vi "Prepare_outputfiles.vi"(8 "error in":errorcluster, 10 "Dynamic data in":T1, 11 "Input parameters 2":T2={"Measurement type"=enum."Debug", "Sensor type"=enum."HPK_8in_256", "Identifier"="test.txt", "Open after execution?"=FALSE, "Plot after execution?"=FALSE, "Display channel"=0, "Voltage Delay (s)"=0.5, "Switch Delay (s)"=0.01, "VISA resource name source"="", "VISA resource name DMM"="", "VISA resource name LCR"="", "Compliance  Level (uA)"=10.0, "Voltage Limit (V)"=1000.0, "Data storage location"="", "Scan voltages"="", "Use source as DMM?"=FALSE, "LCR signal frequenzy (Hz)"=10.0, "DMM device"=enum."Keithley2001", "Sampling number"=1, "Use env. sensors on"=enum."Sensirion sht1x/7x", "Switchboard Handle"=0, "Use Switchboard"=FALSE, "LCR signal voltage (V)"=10000.0, "Repeat"=1, "Test Run Limit (nA)"=10.0, "Scan voltages IV"="", "Scan voltages CV"="", "Hex pad numbers?"=FALSE, "Set measurement type"=enum."Debug", "Custom pad scan"="", "IV voltage Delay (s)"=0.5, "CV voltage Delay (s)"=0.5} {"CV voltage Delay (s)" format="%#_13g"; "IV voltage Delay (s)" format="%#_13g"; "Voltage Limit (V)" format="%#_13g"; "Voltage Delay (s)" format="%#_13g"; "Switch Delay (s)" format="%#_13g"}) -> (0 "error out":errorcluster, 2 "Dynamic data out":T1, 3 "Input parameters":T2={"Measurement type"=enum."Debug", "Sensor type"=enum."HPK_8in_256", "Identifier"="test.txt", "Open after execution?"=FALSE, "Plot after execution?"=FALSE, "Display channel"=0, "Voltage Delay (s)"=0.5, "Switch Delay (s)"=0.01, "VISA resource name source"="", "VISA resource name DMM"="", "VISA resource name LCR"="", "Compliance  Level (uA)"=10.0, "Voltage Limit (V)"=1000.0, "Data storage location"="", "Scan voltages"="", "Use source as DMM?"=FALSE, "LCR signal frequenzy (Hz)"=10.0, "DMM device"=enum."Keithley2001", "Sampling number"=1, "Use env. sensors on"=enum."Sensirion sht1x/7x", "Switchboard Handle"=0, "Use Switchboard"=FALSE, "LCR signal voltage (V)"=10000.0, "Repeat"=1, "Test Run Limit (nA)"=10.0, "Scan voltages IV"="", "Scan voltages CV"="", "Hex pad numbers?"=FALSE, "Set measurement type"=enum."Debug", "Custom pad scan"="", "IV voltage Delay (s)"=0.5, "CV voltage Delay (s)"=0.5} {"CV voltage Delay (s)" format="%#_13g"; "IV voltage Delay (s)" format="%#_13g"; "Voltage Limit (V)" format="%#_13g"; "Voltage Delay (s)" format="%#_13g"; "Switch Delay (s)" format="%#_13g"})   [LabVIEW 2016]
uses:
  Input_parameters.ctl
  Dynamic_data.ctl
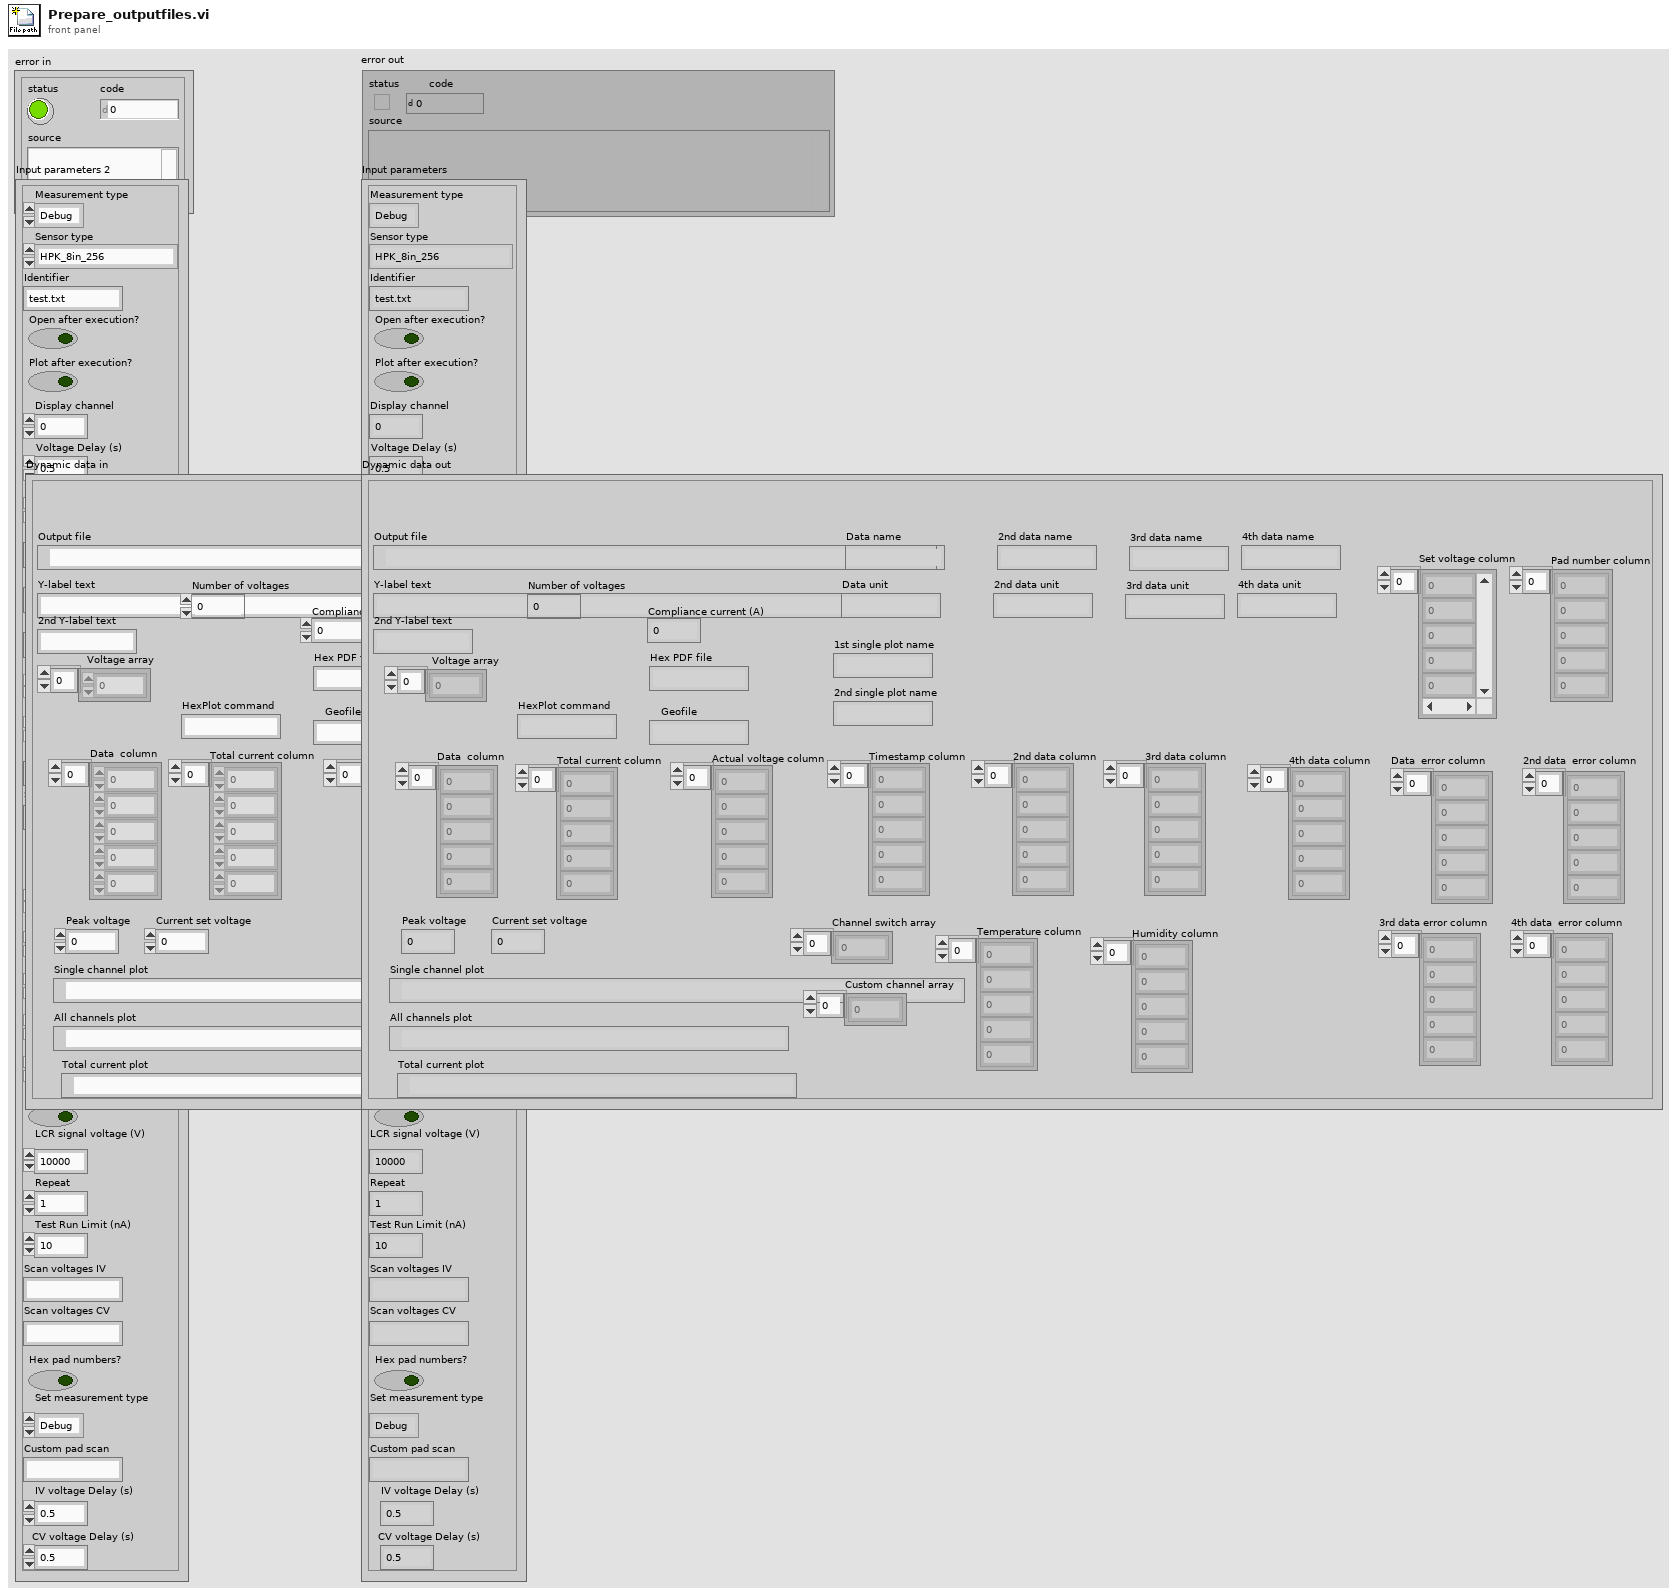
[diagram p1: front panel]
types:
  T1 = typedef "Dynamic_data.ctl" = cluster{"Output file":path, "Y-label text":string, "Current set voltage":dbl, "Set voltage column":dbl[], "Pad number column":dbl[], "Data  column":dbl[], "Number of voltages":i32, "Compliance current (A)":dbl, "Geofile":string, "Peak voltage":dbl, "Hex PDF file":string, "Voltage array":dbl[], "Total current column":dbl[], "Timestamp column":dbl[], "Data name":string, "Data unit":string, "2nd data column":dbl[], "2nd data name":string, "2nd data unit":string, "3rd data column":dbl[], "4th data column":dbl[], "3rd data name":string, "3rd data unit":string, "4th data name":string, "4th data unit":string, "Actual voltage column":dbl[], "2nd Y-label text":string, "Single channel plot":path, "Temperature column":dbl[], "Humidity column":dbl[], "Channel switch array":i32[], "1st single plot name":string, "2nd single plot name":string, "All channels plot":path, "HexPlot command":string, "Custom channel array":i32[], "Data  error column":dbl[], "2nd data  error column":dbl[], "3rd data error column":dbl[], "4th data  error column":dbl[], "Total current plot":path}
  T2 = typedef "Input_parameters.ctl" = cluster{"Measurement type":enum16{"IV", "CV", "Debug", "Test"}, "Sensor type":enum16{"HPK_6in_135", "HPK_8in_256", "INF_8in_256", "Diode", "HPK_6in_256", "Test capacitances", "Full matrix"}, "Identifier":string, "Open after execution?":bool, "Plot after execution?":bool, "Display channel":i32, "Voltage Delay (s)":dbl, "Switch Delay (s)":dbl, "VISA resource name source":refnum<visa-resource-name>, "VISA resource name DMM":refnum<visa-resource-name>, "VISA resource name LCR":refnum<visa-resource-name>, "Compliance  Level (uA)":dbl, "Voltage Limit (V)":dbl, "Data storage location":string, "Scan voltages":string, "Use source as DMM?":bool, "LCR signal frequenzy (Hz)":dbl, "DMM device":enum16{"Keithley2001", "Keithley2450", "Keithley2410", "Keithley6487"}, "Sampling number":i32, "Use env. sensors on":enum16{"Sensirion sht1x/7x", "Switch Matrix", "Probecard"}, "Switchboard Handle":u32, "Use Switchboard":bool, "LCR signal voltage (V)":dbl, "Repeat":i32, "Test Run Limit (nA)":dbl, "Scan voltages IV":string, "Scan voltages CV":string, "Hex pad numbers?":bool, "Set measurement type":enum16{"IV", "CV", "Debug", "Test", "IV+CV"}, "Custom pad scan":string, "IV voltage Delay (s)":dbl, "CV voltage Delay (s)":dbl}
  T3 = enum16{"HPK_6in_135", "HPK_8in_256", "INF_8in_256", "Diode", "HPK_6in_256", "Test capacitances", "Full matrix"}
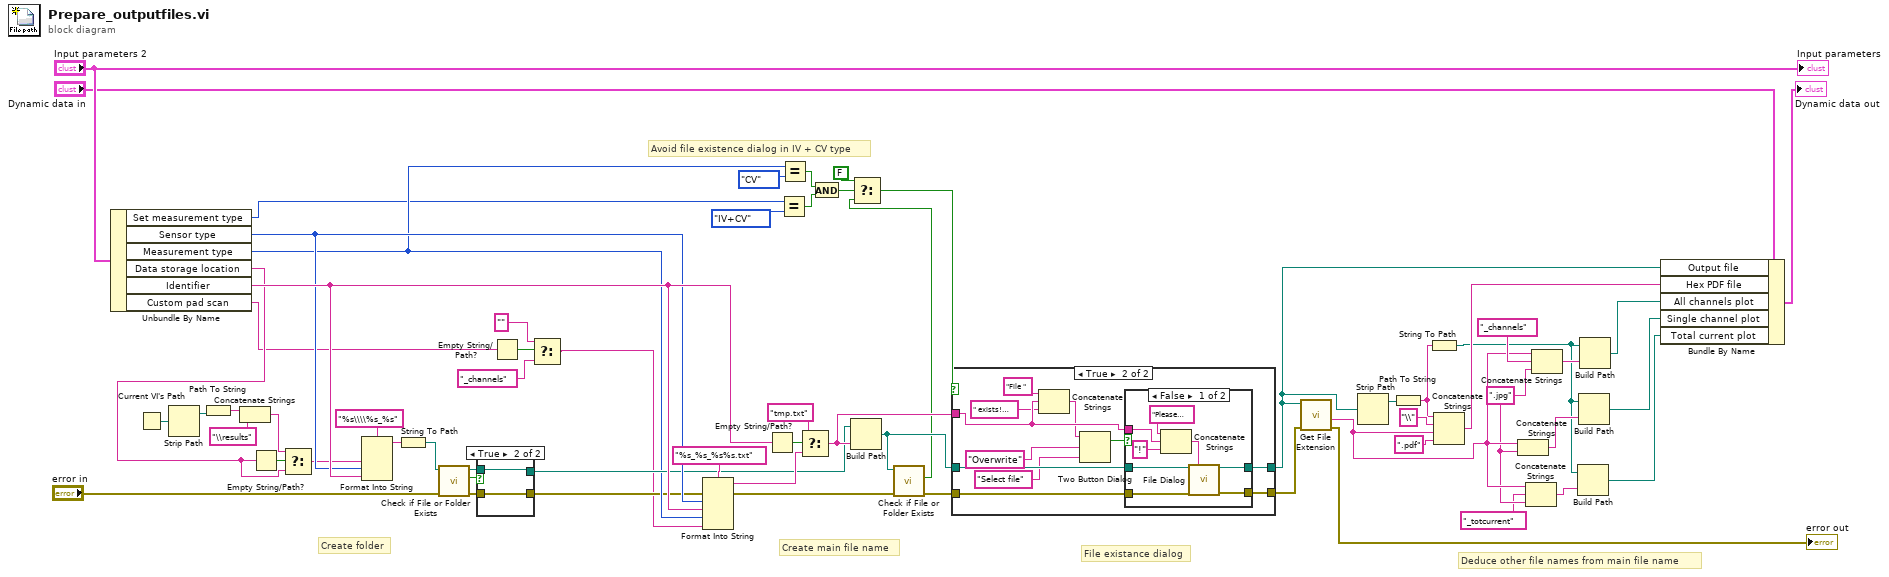
[diagram p0: block diagram]
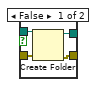
[diagram p2: hidden frame]
diagram:
  w3 = ".jpg" ("string")
  # "Deduce other file names from main file name"
  # "File existance dialog"
  # "Create main file name"
  # "Create folder"
  # "Avoid file existence dialog in IV + CV type"
  n1 = Unbundle By Name("Input parameters 2") -> ("Set measurement type"=w17:enum16{"IV", "CV", "Debug", "Test", "IV+CV"}, "Sensor type"=w37:T3, "Measurement type"=w29:enum16{"IV", "CV", "Debug", "Test"}, "Data storage location"=w13:string, "Identifier"=w38:string, "Custom pad scan"=w11:string)
  n2 = Current VI's Path() -> (path=w60:path)
  n3 = Strip Path(path=w60) -> (stripped path=w59:path)  [unwired: 1 out]
  n4 = Path To String(path=w59) -> (string=w58:string)
  n5 = Concatenate Strings(w58, "\\results" ("string")) -> (w56:string)
  n6 = Empty String/Path?(string/path=w13) -> (empty?=w61:bool)
  n7 = Select(t=w56, s=w61, f=w13) -> (s? t:f=w36:string)
  n8 = Format Into String(format string="%s\\\\%s_%s", w36, w37, w38) -> (resulting string=w35:string)  [unwired: 2 in, 1 out]
  n9 = String To Path(string=w35) -> (path=w33:path)
  n10 = call <vilib>:"Check if File or Folder Exists.vi"("error in (no error)"="error in", "path"=w33) -> ("error out"=w16:errorcluster, "file or folder exists?"=w32:bool, "dup path"=w31:path)  [unwired: 7 in]
  n11 = case shown="True" w32 {
    tunnel: w31 -> [w68 w70]
    tunnel: [w67 w70] -> w30
    tunnel: w16 -> [w66 w69]
    tunnel: [w65 w69] -> w14
    frame False {
      n12 = Create Folder(path (use dialog)=w68, error in=w66) -> (created path=w67:path, error out=w65:errorcluster)  [unwired: 1 in, 1 out]
    }
    frame True {
    }
  }
  n13 = Empty String/Path?(string/path=w11) -> (empty?=w10:bool)
  n14 = Select(t="" ("format string"), s=w10, f="_channels" ("format string")) -> (s? t:f=w7:string)
  n15 = Format Into String(format string="%s_%s_%s%s.txt", error in=w14, w37, w38, w29, w7) -> (resulting string=w52:string, error out=w39:errorcluster)  [unwired: 1 in]
  n16 = Empty String/Path?(string/path=w38) -> (empty?=w55:bool)
  n17 = Equal?(x=w17, y=enum16{"IV", "CV", "Debug", "Test", "IV+CV"}."IV+CV") -> (x = y?=w25:bool)
  n18 = Equal?(x=w29, y=enum16{"IV", "CV", "Debug", "Test"}."CV") -> (x = y?=w24:bool)
  n19 = Select(t="tmp.txt", s=w55, f=w52) -> (s? t:f=w49:string)
  n20 = And(x=w24, y=w25) -> (x .and. y?=w26:bool)
  n21 = Build Path(base path=w30, name or relative path=w49) -> (appended path=w51:path)
  n22 = call <vilib>:"Check if File or Folder Exists.vi"("error in (no error)"=w39, "path"=w51) -> ("error out"=w50:errorcluster, "file or folder exists?"=w22:bool)  [unwired: 7 in, 1 out]
  n23 = Select(t=FALSE, s=w26, f=w22) -> (s? t:f=w21:bool)
  n24 = case shown="True" w21 {
    tunnel: w51 -> [w72 w83]
    tunnel: [w72 w82] -> w48
    tunnel: w50 -> [w71 w81]
    tunnel: [w71 w80] -> w44
    tunnel: w49 -> [_ w79]
    frame False {
    }
    frame True {
      n25 = Concatenate Strings("File " ("string"), w79, " exists! Overwite?" ("string")) -> (w76:string)
      n26 = Two Button Dialog(message=w76, 1:"Select file" ("Center Button Text (\"No\")"), 2:"Overwrite" ("Left Button Text (\"Yes\")")) -> (T button?=w73:bool)
      n27 = case shown="False" w73 {
        tunnel: w83 -> [w91 w93]
        tunnel: [w90 w93] -> w82
        tunnel: w81 -> [w89 w92]
        tunnel: [w88 w92] -> w80
        tunnel: w79 -> [w85 _]
        frame False {
          n28 = Concatenate Strings("Please chose a new file instead of  " ("prompt (Choose or enter file path)"), w85, "!" ("string")) -> (w87:string)
          n29 = call "File Dialog"("start path"=w91, "prompt"=w87, "error in"=w89) -> ("selected path"=w90:path, "error out"=w88:errorcluster)  [unwired: 9 in, 2 out]
        }
        frame True {
        }
      }
    }
  }
  n30 = call <vilib>:"Get File Extension.vi"("error in (no error)"=w44, "file"=w48) -> ("error out"=→"error out":errorcluster, "filename without extension"=w4:string)  [unwired: 5 in, 3 out]
  n31 = Strip Path(path=w48) -> (stripped path=w63:path)  [unwired: 1 out]
  n32 = Path To String(path=w63) -> (string=w45:string)
  n33 = String To Path(string=w45) -> (path=w6:path)
  n34 = Concatenate Strings(w45, "\\" ("string"), w4, ".pdf" ("string")) -> (w47:string)
  n35 = Concatenate Strings(w4, w3) -> (w46:string)
  n36 = Concatenate Strings(w4, "_totcurrent" ("string"), w3) -> (w5:string)
  n37 = Concatenate Strings(w4, "_channels" ("string"), w3) -> (w43:string)
  n38 = Build Path(base path=w6, name or relative path=w5) -> (appended path=w1:path)
  n39 = Build Path(base path=w6, name or relative path=w46) -> (appended path=w41:path)
  n40 = Build Path(base path=w6, name or relative path=w43) -> (appended path=w40:path)
  n41 = Bundle By Name(cluster="Dynamic data in", "Output file"=w48, "Hex PDF file"=w47, "All channels plot"=w40, "Single channel plot"=w41, "Total current plot"=w1) -> (→"Dynamic data out":T1)
  "Input parameters" <- "Input parameters 2"
